vi "Get ECAT IOVar Data.vi"(8 "Fehler (Eingang, kein Fehler)":errorcluster, 10 "ECAT Variablenobjekt":refnum<k21>[](array[refnum]), 11 "VS ref":T5=18446744073709551615 format="%.0x") -> (0 "Fehler (Ausgang)":errorcluster, 1 "I/O Output Vars":T6[](array[typedef]) {"VS ref" format="%.0x"}, 2 "I/O Imput Vars":T6[](array[typedef]) {"VS ref" format="%.0x"}, 3 "VS ref 2":T5=18446744073709551615 format="%.0x", 5 "I/O Output Data":T1 {"BD Refs"."Data Reference" format="%.0x"}, 7 "I/O Input Data":T4 {"BD Refs"."Data Reference" format="%.0x"})   [LabVIEW 2015, in "Scan Engine Custom Device.lvlib"]
uses:
  Scan Engine Custom Device.lvlib
  Type Defs/Generic ECAT Slave IOV Cluster.ctl
  <vilib>/NI Veristand/Custom Device API/Custom Device Item Ref.ctl
  Type Defs/UDV Data Type.ctl
  Type Defs/Input Data.ctl
  <vilib>/NI Veristand/Custom Device API/Block Data Reference.ctl
  <vilib>/NI Veristand/Custom Device API/Data Reference.ctl
  Type Defs/Output Data.ctl
  <vilib>/NI Veristand/Custom Device API/Data Access Type.ctl
  Type Defs/Data Ref FGV Command.ctl
  Globals/Property Strings.vi
  <vilib>/NI Veristand/Custom Device API/Custom Device API.lvlib
  <resource>/objmgr/ni.var.rc
panel:
  out "ECAT Variablenobjekt out":refnum<k21>[](array[refnum])
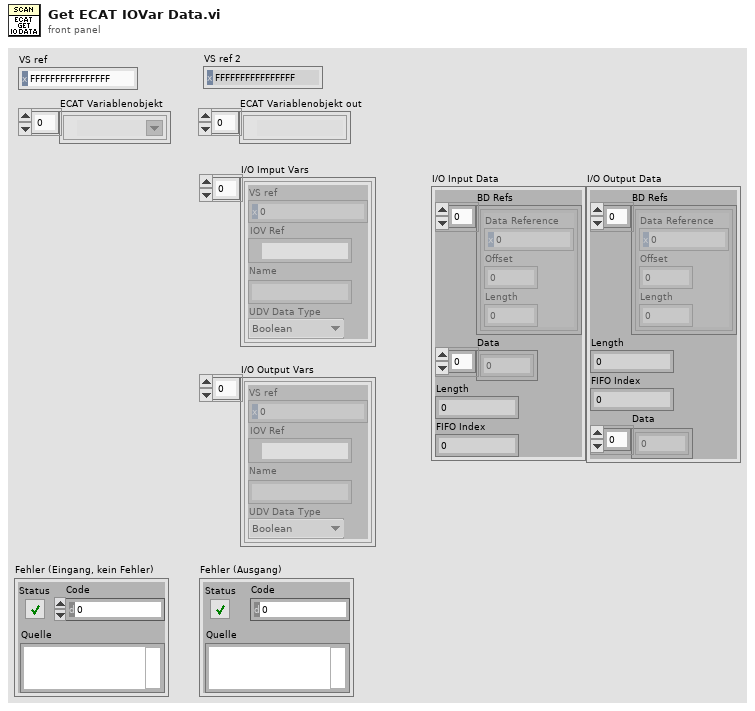
[diagram p1: front panel]
types:
  T1 = typedef "Scan Engine Custom Device.lvlib/Output Data.ctl" = cluster{"BD Refs":T2[], "Length":i32, "FIFO Index":i32, "Data":dbl[]}
  T2 = typedef "Custom Device API.lvlib/Block Data Reference.ctl" = cluster{"Data Reference":T3, "Offset":u64, "Length":u64}
  T3 = typedef "Custom Device API.lvlib/Data Reference.ctl" = i32
  T4 = typedef "Scan Engine Custom Device.lvlib/Input Data.ctl" = cluster{"BD Refs":T2[], "Data":dbl[], "Length":i32, "FIFO Index":i32}
  T5 = typedef "Custom Device API.lvlib/Custom Device Item Ref.ctl" = u64
  T6 = typedef "Scan Engine Custom Device.lvlib/Generic ECAT Slave IOV Cluster.ctl" = cluster{"VS ref":T5, "IOV Ref":refnum<k21>, "Name":string, "UDV Data Type":T7}
  T7 = typedef "Scan Engine Custom Device.lvlib/UDV Data Type.ctl" = enum16{"Boolean", "Fixed Point", "Int8", "Int16", "Int32", "Int64", "U32 Bit Field", "UInt8", "UInt16", "UInt32", "UInt64", "Other"}
  T8 = typedef "Scan Engine Custom Device.lvlib/Data Ref FGV Command.ctl" = enum16{"Intialize", "Get", "Update"}
  T9 = typedef "Custom Device API.lvlib/Data Access Type.ctl" = enum16{"Read", "Write"}
  T10 = typedef "Scan Engine Custom Device.lvlib/ECAT Channel Data Type.ctl" = enum16{"Boolean", "Fixed Point", "Int8", "Int16", "Int32", "Int64", "U32 Bit Field", "UInt8", "UInt16", "UInt32", "UInt64", "Other", "DBL"}
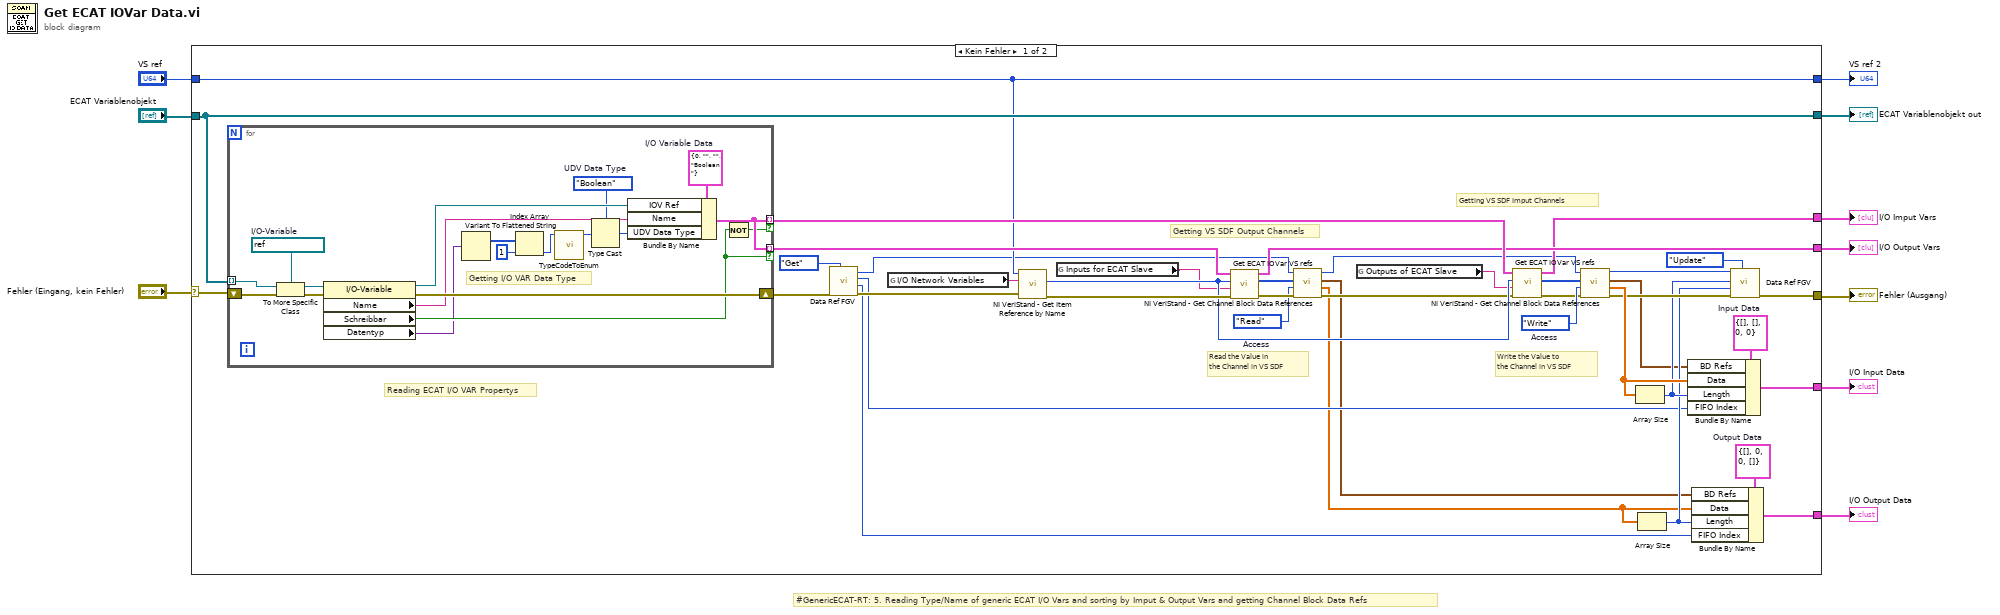
[diagram p0: block diagram]
diagram:
  # "#GenericECAT-RT: 5. Reading Type/Name of generic ECAT I/O Vars and sorting by Imput & Output Vars and getting Channel Block Data Refs"
  n1 = case shown="Kein Fehler" "Fehler (Eingang, kein Fehler)" {
    selector: "Fehler (Eingang, kein Fehler)" -> [w48 w72]
    tunnel: "ECAT Variablenobjekt" -> [w50 w71]
    tunnel: [w26 w72] -> w8
    tunnel: [w50 w71] -> w7
    tunnel: "VS ref" -> [w36 w70]
    tunnel: [w44 _] -> w5
    tunnel: [w43 _] -> w4
    tunnel: [w36 w70] -> w3
    tunnel: [w33 _] -> w2
    tunnel: [w32 _] -> w1
    frame No Error {
      w34 = T1 {"BD Refs"=[], "Length"=0, "FIFO Index"=0, "Data"=[]}  # Output Data
      w35 = T4 {"BD Refs"=[], "Data"=[], "Length"=0, "FIFO Index"=0}  # Input Data
      w38 = Data_Access_Type."Write"  # Access
      w40 = Data_Access_Type."Read"  # Access
      # "Getting VS SDF Imput Channels"
      # "Getting VS SDF Output Channels"
      # "Reading ECAT I/O VAR Propertys"
      # "Write the Value to\nthe Channel in VS SDF"
      # "Read the Value in\nthe Channel in VS SDF"
      n2 = for {
        shift-right: [w69] -> w29
        shift-left: w48 -> [w63]
        tunnel: w50 -> [w62] mode=indexing
        tunnel: [w66] -> w45 mode=indexing if=w65
        tunnel: [w66] -> w49 mode=indexing if=w64
        w54 = UDV_Data_Type."Boolean"  # UDV Data Type
        w61 = refnum<k21> refnum  # I/O-Variable
        w68 = T6 {"VS ref"=0, "IOV Ref"="", "Name"="", "UDV Data Type"=enum."Boolean"}  # I/O Variable Data
        # "Getting I/O VAR Data Type"
        n3 = To More Specific Class(target class=w61, reference=w62, error in=w63) -> (specific class reference=w60:refnum<k21>, error out=w59:errorcluster)
        n4 = property class="I/O-Variable"(reference=w60, error in=w59) -> (reference out=w67:refnum<k21>, error out=w69:errorcluster, "Name"=w52:string, "Schreibbar"=w64:bool, "Datentyp"=w56:variant)
        n5 = Variant To Flattened String(Variant=w56) -> (1:w57:i16[])  [unwired: 1 out]
        n6 = Index Array(array=w57, index=1) -> (element=w55:i16)
        n7 = call "TypeCodeToEnum.vi"("Type Code (numbers in hexadecimal)"=w55) -> ("UDV Data Type"=w53:T10)  [unwired: 9 in, 1 out]
        n8 = Type Cast(type=w54, x=w53) -> (*(type *) &x=w51:T7)
        n9 = Bundle By Name(cluster=w68, "IOV Ref"=w67, "Name"=w52, "UDV Data Type"=w51) -> (w66:T6)
        n10 = Not(x=w64) -> (.not. x?=w65:bool)
      }
      n11 = call "Data Ref FGV.vi"("Command"=Data_Ref_FGV_Command."Get", "error in (no error)"=w29) -> ("error out"=w28:errorcluster, "Output FIFO Index / Length"=w19:i32, "Input FIFO Index / Length"=w18:i32, "Device Ref out"=w13:T5)  [unwired: 6 in]
      n12 = global read "Property Strings.vi" "I/O Network Variables"() -> (w47:string)
      n13 = call <vilib>:"NI VeriStand - Get Item Reference by Name.vi"("error in (no error)"=w28, "Item Name"=w47, "Parent Ref in"=w36) -> ("error out"=w46:errorcluster, "Item Ref"=w42:T5)  [unwired: 5 in, 2 out]
      n14 = global read "Property Strings.vi" "Inputs for ECAT Slave"() -> (w23:string)
      n15 = call "Get ECAT IOVar VS refs.vi"("Fehler (Eingang, kein Fehler)"=w46, "Section Name"=w23, "Item Ref"=w42, "I/O Variable Data in"=w49) -> ("Fehler (Ausgang)"=w41:errorcluster, "Channel Refs"=w11:T5[], "I/O Variable Data out"=w44:T6[])  [unwired: 5 in]
      n16 = call <vilib>:"NI VeriStand - Get Channel Block Data References.vi"("error in (no error)"=w41, "Access"=w40, "Channel Refs"=w11, "Device Ref in"=w13) -> ("error out"=w39:errorcluster, "Values Array"=w17:dbl[], "Block Data Refs"=w15:T2[], "Device Ref out"=w14:T5)  [unwired: 4 in]
      n17 = global read "Property Strings.vi" "Outputs of ECAT Slave"() -> (w22:string)
      n18 = call "Get ECAT IOVar VS refs.vi"("Fehler (Eingang, kein Fehler)"=w39, "Section Name"=w22, "Item Ref"=w42, "I/O Variable Data in"=w45) -> ("Fehler (Ausgang)"=w37:errorcluster, "Channel Refs"=w12:T5[], "I/O Variable Data out"=w43:T6[])  [unwired: 5 in]
      n19 = call <vilib>:"NI VeriStand - Get Channel Block Data References.vi"("error in (no error)"=w37, "Access"=w38, "Channel Refs"=w12, "Device Ref in"=w14) -> ("error out"=w27:errorcluster, "Values Array"=w30:dbl[], "Block Data Refs"=w16:T2[], "Device Ref out"=w24:T5)  [unwired: 4 in]
      n20 = Array Size(array=w30) -> (size(s)=w21:i32)
      n21 = Array Size(array=w17) -> (size(s)=w20:i32)
      n22 = Bundle By Name(cluster=w35, "BD Refs"=w16, "Data"=w30, "Length"=w21, "FIFO Index"=w18) -> (w33:T4)
      n23 = Bundle By Name(cluster=w34, "BD Refs"=w15, "Data"=w17, "Length"=w20, "FIFO Index"=w19) -> (w32:T1)
      n24 = call "Data Ref FGV.vi"("Command"=Data_Ref_FGV_Command."Update", "error in (no error)"=w27, "Output Length"=w20, "Input Length"=w21, "Device Ref in"=w24) -> ("error out"=w26:errorcluster)  [unwired: 3 in, 3 out]
    }
    frame Error {
    }
  }
  "I/O Imput Vars" <- w4
  "I/O Output Vars" <- w5
  "Fehler (Ausgang)" <- w8
  "ECAT Variablenobjekt out" <- w7
  "VS ref 2" <- w3
  "I/O Input Data" <- w2
  "I/O Output Data" <- w1
